vi "CommandList.vi"(0 "DashboardServer.lvclass":refnum<class "Universal Robot.lvclass">) -> (14 "DashboardServer.lvclass out":refnum<class "Universal Robot.lvclass">, 19 "Compatible Commands":T1[](array[typedef])=[{"Command"="Load", "Input"=FALSE, "Input Type"="", "Remote Mode Required"=FALSE, "Min Version"={"Major"=0, "Minor"=0, "Fix"=0, "Build"=0}, "Deprecated"=FALSE}, {"Command"="Play", "Input"=FALSE, "Input Type"="", "Remote Mode Required"=FALSE, "Min Version"={"Major"=0, "Minor"=0, "Fix"=0, "Build"=0}, "Deprecated"=FALSE}, {"Command"="Stop", "Input"=FALSE, "Input Type"="", "Remote Mode Required"=FALSE, "Min Version"={"Major"=0, "Minor"=0, "Fix"=0, "Build"=0}, "Deprecated"=FALSE}, {"Command"="Pause", "Input"=FALSE, "Input Type"="", "Remote Mode Required"=FALSE, "Min Version"={"Major"=0, "Minor"=0, "Fix"=0, "Build"=0}, "Deprecated"=FALSE}, {"Command"="Quit", "Input"=FALSE, "Input Type"="", "Remote Mode Required"=FALSE, "Min Version"={"Major"=0, "Minor"=0, "Fix"=0, "Build"=0}, "Deprecated"=FALSE}, {"Command"="Shutdown", "Input"=FALSE, "Input Type"="", "Remote Mode Required"=FALSE, "Min Version"={"Major"=0, "Minor"=0, "Fix"=0, "Build"=0}, "Deprecated"=FALSE}, {"Command"="Running", "Input"=FALSE, "Input Type"="", "Remote Mode Required"=FALSE, "Min Version"={"Major"=0, "Minor"=0, "Fix"=0, "Build"=0}, "Deprecated"=FALSE}, {"Command"="Robotmode", "Input"=FALSE, "Input Type"="", "Remote Mode Required"=FALSE, "Min Version"={"Major"=0, "Minor"=0, "Fix"=0, "Build"=0}, "Deprecated"=FALSE}, {"Command"="get loaded program", "Input"=FALSE, "Input Type"="", "Remote Mode Required"=FALSE, "Min Version"={"Major"=0, "Minor"=0, "Fix"=0, "Build"=0}, "Deprecated"=FALSE}, {"Command"="popup", "Input"=TRUE, "Input Type"="<popup-text>", "Remote Mode Required"=FALSE, "Min Version"={"Major"=0, "Minor"=0, "Fix"=0, "Build"=0}, "Deprecated"=FALSE}, {"Command"="close popup", "Input"=FALSE, "Input Type"="", "Remote Mode Required"=FALSE, "Min Version"={"Major"=0, "Minor"=0, "Fix"=0, "Build"=0}, "Deprecated"=FALSE}, {"Command"="addToLog", "Input"=FALSE, "Input Type"="<log-message>", "Remote Mode Required"=FALSE, "Min Version"={"Major"=0, "Minor"=0, "Fix"=0, "Build"=0}, "Deprecated"=FALSE}, {"Command"="IsProgramSaved", "Input"=FALSE, "Input Type"="", "Remote Mode Required"=FALSE, "Min Version"={"Major"=0, "Minor"=0, "Fix"=0, "Build"=0}, "Deprecated"=FALSE}, {"Command"="programState", "Input"=FALSE, "Input Type"="", "Remote Mode Required"=FALSE, "Min Version"={"Major"=0, "Minor"=0, "Fix"=0, "Build"=0}, "Deprecated"=FALSE}, {"Command"="PolyscopeVersion", "Input"=FALSE, "Input Type"="", "Remote Mode Required"=FALSE, "Min Version"={"Major"=0, "Minor"=0, "Fix"=0, "Build"=0}, "Deprecated"=FALSE}, {"Command"="set operational mode", "Input"=FALSE, "Input Type"="<mode>", "Remote Mode Required"=FALSE, "Min Version"={"Major"=0, "Minor"=0, "Fix"=0, "Build"=0}, "Deprecated"=FALSE}, {"Command"="clear operational mode", "Input"=FALSE, "Input Type"="", "Remote Mode Required"=FALSE, "Min Version"={"Major"=0, "Minor"=0, "Fix"=0, "Build"=0}, "Deprecated"=FALSE}, {"Command"="power on", "Input"=FALSE, "Input Type"="", "Remote Mode Required"=FALSE, "Min Version"={"Major"=0, "Minor"=0, "Fix"=0, "Build"=0}, "Deprecated"=FALSE}, {"Command"="power off", "Input"=FALSE, "Input Type"="", "Remote Mode Required"=FALSE, "Min Version"={"Major"=0, "Minor"=0, "Fix"=0, "Build"=0}, "Deprecated"=FALSE}])   [LabVIEW 2019, in "Universal Robot.lvclass"]
uses:
  Universal Robot.lvclass
  PolyScopeCommand.ctl
  PolyScopeVersion.ctl
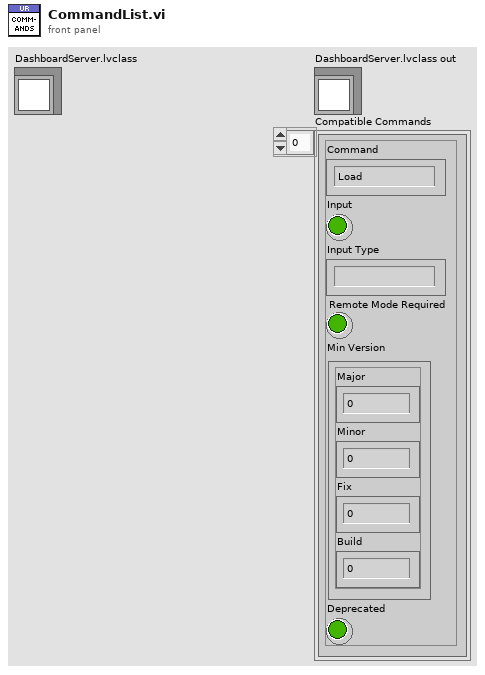
[diagram p1: front panel]
types:
  T1 = typedef "Universal Robot.lvclass/PolyScopeCommand.ctl" = cluster{"Command":string, "Input":bool, "Input Type":string, "Remote Mode Required":bool, "Min Version":T2, "Deprecated":bool}
  T2 = typedef "Universal Robot.lvclass/PolyScopeVersion.ctl" = cluster{"Major":i32, "Minor":i32, "Fix":i32, "Build":i32}
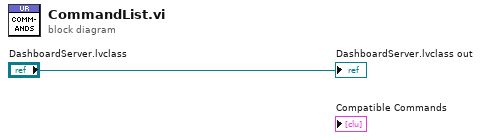
[diagram p0: block diagram]
diagram:
  "DashboardServer.lvclass out" <- "DashboardServer.lvclass"
